vi "Initialize.vi"(6 "Allow go to default? (True)":bool=TRUE, 8 "error in (no error)":errorcluster, 9 "Reset (True)":bool=TRUE, 10 "ID Query (True)":bool=TRUE, 11 "VISA resource name":refnum<visa-resource-name>) -> (0 "error out":errorcluster, 2 "idn string":string, 3 "VISA resource name out":refnum<visa-resource-name>)   [LabVIEW 2020, in "3458A Basic Driver.lvlib"]
doc: "Establishes communication with the instrument and optionally performs an instrument identification query and/or an instrument reset. It also places the instrument in a default state needed for other instrument driver operations. Therefore, call this VI before calling other instrument driver VIs for this instrument. Generally, you need to call the Initialize VI only once at the beginning of an application."
uses:
  3458A Basic Driver.lvlib
panel:
  # "(c) 2007  National Instruments.  ALL RIGHTS RESERVED."
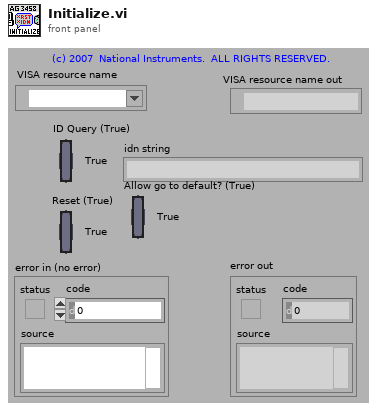
[diagram p1: front panel]
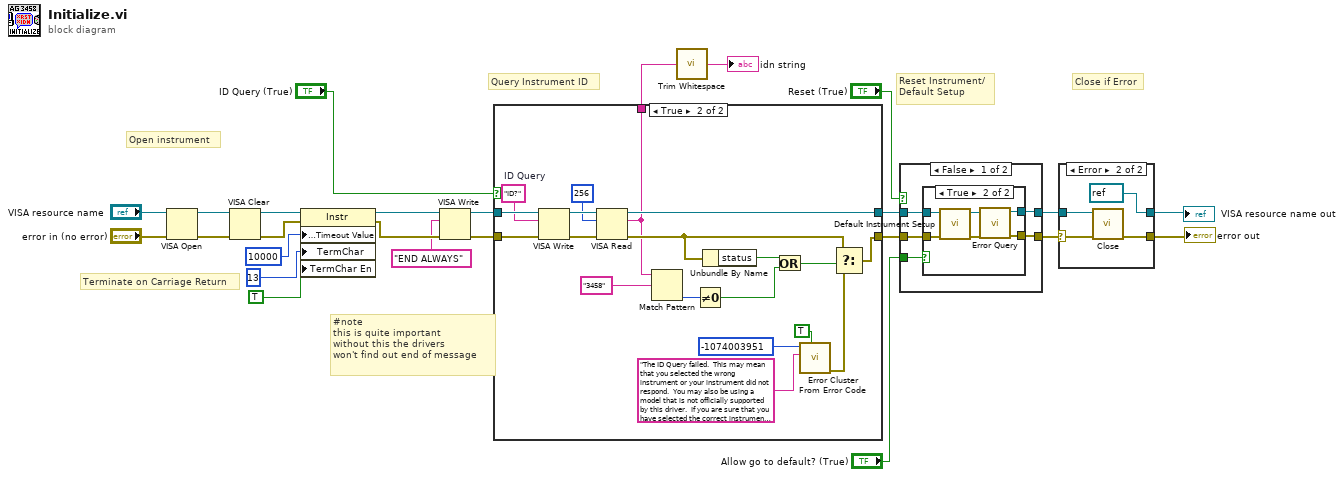
[diagram p0: block diagram]
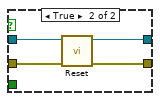
[diagram p4: hidden frame]
diagram:
  # "#note\nthis is quite important\nwithout this the drivers\nwon't find out end of message"
  # "Terminate on Carriage Return"
  # "Close if Error"
  # "Query Instrument ID"
  # "Reset Instrument/\nDefault Setup"
  # "Open instrument"
  n1 = VISA Open(error in (no error)="error in (no error)", VISA resource name="VISA resource name") -> (VISA resource name=w21:refnum<visa-resource-name>, error out=w20:errorcluster)  [unwired: 3 in]
  n2 = VISA Clear(VISA resource name=w21, error in (no error)=w20) -> (VISA resource name out=w19:refnum<visa-resource-name>, error out=w18:errorcluster)
  n3 = property class="Instr"(reference=w19, error in=w18, "General Settings:Timeout Value"=u32 10000, "TermChar"=u8 13 ("Message Based Settings:Termination Character"), "TermChar En"=TRUE ("Message Based Settings:Termination Character Enable")) -> (reference out=w4:refnum<visa-resource-name>, error out=w3:errorcluster)
  n4 = VISA Write(VISA resource name=w4, write buffer="END ALWAYS", error in (no error)=w3) -> (VISA resource name out=w5:refnum<visa-resource-name>, error out=w6:errorcluster)  [unwired: 1 out]
  n5 = case shown="True" "ID Query (True)" {
    tunnel: [w26 w46] -> w24
    tunnel: [w27 w43] -> w25
    tunnel: w5 -> [w27 w44]
    tunnel: w6 -> [w26 w45]
    tunnel: [_ w28] -> w8
    frame False {
    }
    frame True {
      w38 = "ID?"  # ID Query
      n6 = VISA Write(VISA resource name=w44, write buffer=w38, error in (no error)=w45) -> (VISA resource name out=w42:refnum<visa-resource-name>, error out=w41:errorcluster)  [unwired: 1 out]
      n7 = VISA Read(VISA resource name=w42, byte count=u32 256, error in (no error)=w41) -> (VISA resource name out=w43:refnum<visa-resource-name>, read buffer=w28:string, error out=w32:errorcluster)  [unwired: 1 out]
      n8 = Match Pattern(string=w28, regular expression="3458") -> (offset past match=w33:i32)  [unwired: 1 in, 3 out]
      n9 = Not Equal To 0?(x=w33) -> (x != 0?=w29:bool)
      n10 = Unbundle By Name(w32) -> ("status"=w31:bool)
      n11 = Or(x=w31, y=w29) -> (x .or. y?=w30:bool)
      n12 = call <vilib>:"Error Cluster From Error Code.vi"("show call chain? (False)"=TRUE, "error message (\"\")"="The ID Query failed.  This may mean that you selected the wrong instrument or your instrument did not respond.  You may also be using a model that is not officially supported by this driver.  If you are sure that you have selected the correct instrument and it is responding, try disabling the ID Query." ("Source (VI Name)"), "error code (0)"=-1074003951 ("Code")) -> ("error out"=w37:errorcluster)  [unwired: 6 in]
      n13 = Select(t=w32, s=w30, f=w37) -> (s? t:f=w46:errorcluster)
    }
  }
  n14 = call <vilib>:"Trim Whitespace.vi"("string"=w8) -> ("trimmed string"=→"idn string":string)  [unwired: 1 in]
  n15 = case shown="False" "Reset (True)" {
    tunnel: w24 -> [w50 w61]
    tunnel: [w48 w60] -> w16
    tunnel: w25 -> [w51 w62]
    tunnel: [w49 w63] -> w17
    tunnel: "Allow go to default? (True)" -> [w47 _]
    frame False {
      n16 = case shown="True" w47 {
        tunnel: w51 -> [w52 w59]
        tunnel: w50 -> [w53 w58]
        tunnel: [w52 w55] -> w49
        tunnel: [w53 w54] -> w48
        frame False {
        }
        frame True {
          n17 = call "Default Instrument Setup.vi"("error in (no error)"=w58, "VISA resource name"=w59) -> ("error out"=w56:errorcluster, "VISA resource name out"=w57:refnum<visa-resource-name>)  [unwired: 8 in]
          n18 = call "Error Query.vi"("error in (no error)"=w56, "VISA resource name"=w57) -> ("error out"=w54:errorcluster, "VISA resource name out"=w55:refnum<visa-resource-name>)  [unwired: 6 in, 2 out]
        }
      }
    }
    frame True {
      n19 = call "Reset.vi"("error in (no error)"=w61, "VISA resource name"=w62) -> ("error out"=w60:errorcluster, "VISA resource name out"=w63:refnum<visa-resource-name>)  [unwired: 8 in]
    }
  }
  n20 = case shown="Error" w16 {
    selector: w16 -> [w64 w67]
    tunnel: w17 -> [w65 w68]
    tunnel: [w65 refnum<visa-resource-name> refnum ("VISA resource name out")] -> w11
    tunnel: [w64 w69] -> w9
    frame No Error {
    }
    frame Error {
      n21 = call "Close.vi"("error in (no error)"=w67, "VISA resource name"=w68) -> ("error out"=w69:errorcluster)  [unwired: 9 in]
    }
  }
  "VISA resource name out" <- w11
  "error out" <- w9
